vi "Open Control Shortcut Menu Reference.vi"(8 "error in (no error)":errorcluster, 11 "IControlShortcutMenu in":refnum<class "IControlShortcutMenu.lvclass">) -> (0 "error out":errorcluster, 3 "Shortcut Menu Reference":T1)   [LabVIEW 2015, in "ActorEvents.lvlib" / "IControlShortcutMenu.lvclass"]
uses:
  IControlShortcutMenu.lvclass
  ControlShortcutMenu Reference.ctl
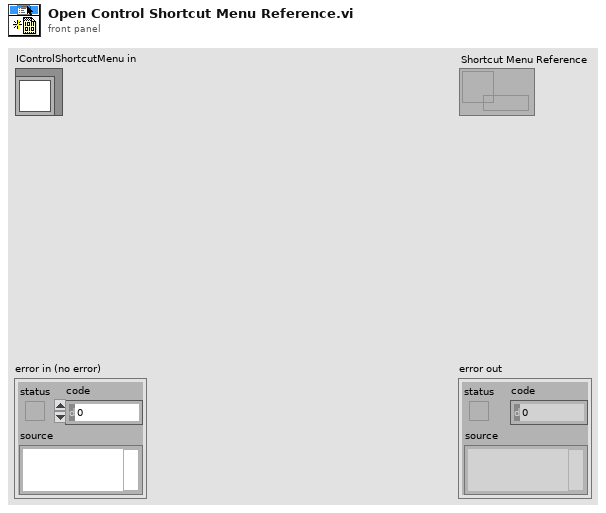
[diagram p1: front panel]
types:
  T1 = typedef "ActorEvents.lvlib/IControlShortcutMenu.lvclass/ControlShortcutMenu Reference.ctl" = refnum<data-value>
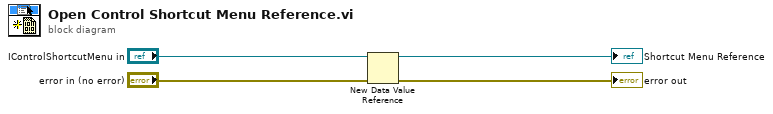
[diagram p0: block diagram]
diagram:
  n1 = New Data Value Reference(data value="IControlShortcutMenu in", error in="error in (no error)") -> (data value reference=→"Shortcut Menu Reference":refnum<data-value>, error out=→"error out":errorcluster)
